vi "DataStream_PC_Close.vi"(8 "Error":errorcluster, 11 "Stream Ref":T1) -> (0 "Error Out":errorcluster)   [LabVIEW 2020]
uses:
  TypeDefs/Cluster_DataStream_PC Reader Refs.ctl
  <vilib>/ErrorRing/Error Ring.xnode
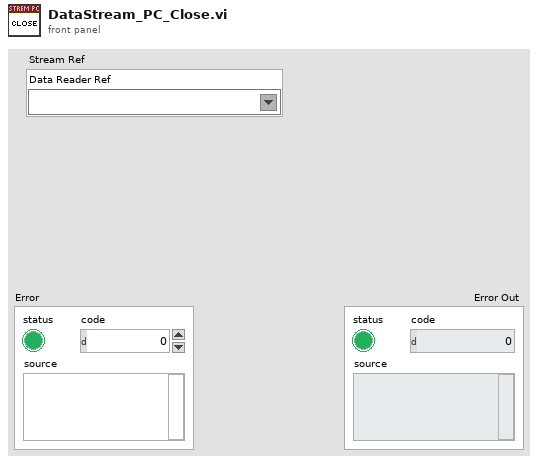
[diagram p1: front panel]
types:
  T1 = typedef "Cluster_DataStream_PC Reader Refs.ctl" = cluster{"Data Reader Ref":refnum<k21>}
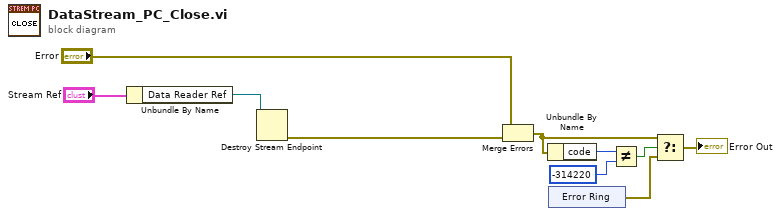
[diagram p0: block diagram]
diagram:
  n1 = Unbundle By Name("Stream Ref") -> ("Data Reader Ref"=w3:refnum<k21>)
  n2 = Destroy Stream Endpoint(11:w3) -> (0:w8:errorcluster)  [unwired: 1 in]
  n3 = Merge Errors("Error", w8) -> (w2:errorcluster)
  n4 = Unbundle By Name(w2) -> ("code"=w5:i32)
  n5 = xnode "Error Ring"() -> ("error out"=w9:errorcluster)
  n6 = Not Equal?(x=w5, y=-314220) -> (x != y?=w7:bool)
  n7 = Select(t=w2, s=w7, f=w9) -> (s? t:f=→"Error Out":errorcluster)
